vi "ProtoDemo.vi"() -> ()   [LabVIEW 2020, in "VolatusScratch.lvlib"]
uses:
  VolatusScratch.lvlib
  messages/StartLog/Data.ctl
  messages/StartLog/StartLog.lvlib
panel:
  out "Buffer":u8[](array[numeric]) format="%.0x"
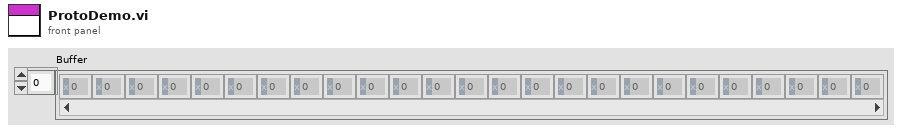
[diagram p1: front panel]
types:
  T1 = typedef "StartLog.lvlib/Data.ctl" = cluster{"series":string, "timestamp":string}
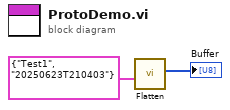
[diagram p0: block diagram]
diagram:
  n1 = call "Flatten.vi"("Data"=T1 {"series"="Test1", "timestamp"="20250623T210403"} ("StartLog")) -> ("Buffer"=→"Buffer":u8[])  [unwired: 9 in, 1 out]
